vi "set Requested Resources property.vi"(8 "error in (no error)":errorcluster, 10 "Requested Resources":T1, 11 "Section Ptr":T4 format="%.0x") -> (0 "error out":errorcluster, 3 "Item Ref out":T4 format="%.0x")   [LabVIEW 2016, in "FPGA RM System Definition API.lvlib"]
uses:
  FPGA RM System Definition API.lvlib
  <vilib>/NI Veristand/Custom Device API/Custom Device Item Ref.ctl
  Shared/FPGA Configuration Classes/Datatype Group/Requested Resources.ctl
  Shared/Types/Requested Resource.ctl
  Shared/Types/Channel Type.ctl
  <vilib>/NI Veristand/Custom Device API/Set Item Property (Variant).vi
  <vilib>/NI VeriStand/Custom Device API/Custom Device API.lvlib
  Shared/FPGA RM Shared API.lvlib
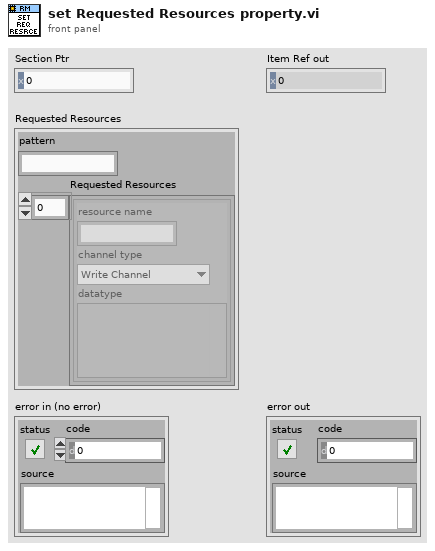
[diagram p1: front panel]
types:
  T1 = typedef "FPGA RM Shared API.lvlib/Requested Resources.ctl" = cluster{"pattern":string, "Requested Resources":T2[]}
  T2 = typedef "FPGA RM Shared API.lvlib/Requested Resource.ctl" = cluster{"resource name":string, "channel type":T3, "datatype":variant}
  T3 = typedef "FPGA RM Shared API.lvlib/Channel Type.ctl" = enum16{"Write Channel", "Read Channel", "Write Waveform", "Read Waveform"}
  T4 = typedef "Custom Device API.lvlib/Custom Device Item Ref.ctl" = u64
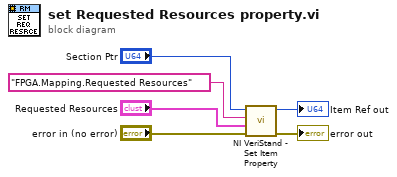
[diagram p0: block diagram]
diagram:
  n1 = call-poly <vilib>:"NI VeriStand - Set Item Property.vi"("error in (no error)"="error in (no error)", "Value"="Requested Resources", "Property Name"="FPGA.Mapping.Requested Resources", "Item Ref in"="Section Ptr") -> ("error out"=→"error out":errorcluster, "Item Ref out"=→"Item Ref out":T4)  [unwired: 5 in, 1 out]
